vi "FreqResolution.vi"(1 "finalSize":i32) -> (0 "frequency":dbl)   [LabVIEW 2011]
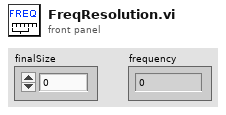
[diagram p1: front panel]
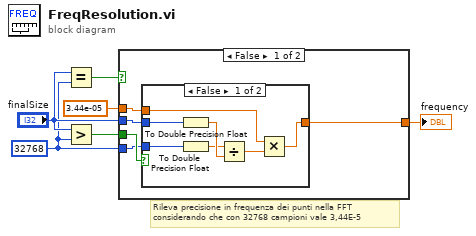
[diagram p0: block diagram]
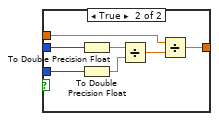
[diagram p2: hidden frame]
diagram:
  w2 = 32768 ("y")
  # "Rileva precisione in frequenza dei punti nella FFT\nconsiderando che con 32768 campioni vale 3,44E-5"
  n1 = Equal?(x="finalSize", y=w2) -> (x = y?=w1:bool)
  n2 = Greater?(x="finalSize", y=w2) -> (0:w3:bool)
  n3 = case shown="False" w1 {
    tunnel: w2 -> [w10 _]
    tunnel: [w7 w26] -> w6
    tunnel: w3 -> [w11 _]
    tunnel: "finalSize" -> [w9 _]
    tunnel: 3.44e-05 ("y") -> [w8 w26]
    frame False {
      n4 = case shown="False" w11 {
        tunnel: w10 -> [w15 w25]
        tunnel: w9 -> [w14 w23]
        tunnel: w8 -> [w13 w21]
        tunnel: [w12 w19] -> w7
        frame False {
          n5 = To Double Precision Float(number=w14) -> (double precision float=w18:dbl)
          n6 = To Double Precision Float(number=w15) -> (double precision float=w17:dbl)
          n7 = Divide(x=w17, y=w18) -> (x/y=w16:dbl)
          n8 = Multiply(x=w13, y=w16) -> (x*y=w12:dbl)
        }
        frame True {
          n9 = To Double Precision Float(number=w23) -> (double precision float=w22:dbl)
          n10 = To Double Precision Float(number=w25) -> (double precision float=w24:dbl)
          n11 = Divide(x=w22, y=w24) -> (x/y=w20:dbl)
          n12 = Divide(x=w21, y=w20) -> (x/y=w19:dbl)
        }
      }
    }
    frame True {
    }
  }
  "frequency" <- w6
